vi "Write From File To Instrument.vi"(8 "error in (no error)":errorcluster, 9 "Target Instrument File":string="D:\\user\\data\\test.hcp", 10 "Source PC File":path=path "C:/test.hcp", 11 "VISA resource name":refnum<visa-resource-name>) -> (0 "error out":errorcluster, 3 "VISA resource name out":refnum<visa-resource-name>)   [LabVIEW 2020, in "Rohde&Schwarz CMXP GPRF.lvlib"]
doc: "This VI copies a file from the host computer to the instrument:\n<b>PC FILE -> INSTRUMENT FILE</b>\n\nRemote-control command:\nMMEMory:DATA <file_name>[,<block data>]"
uses:
  <instrlib>/Rohde&Schwarz CMXP GPRF/Rohde&Schwarz CMXP GPRF.lvlib
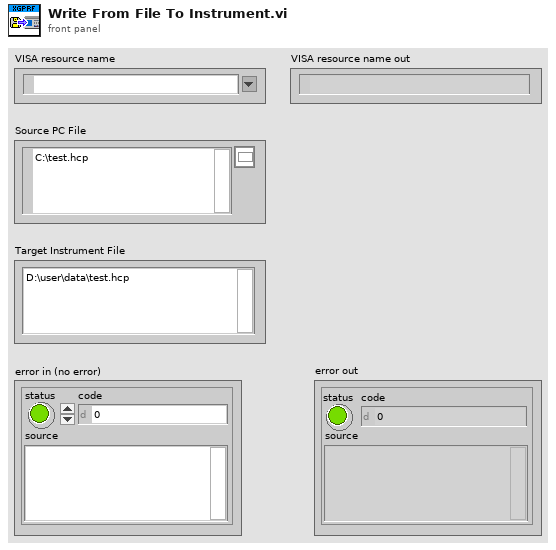
[diagram p1: front panel]
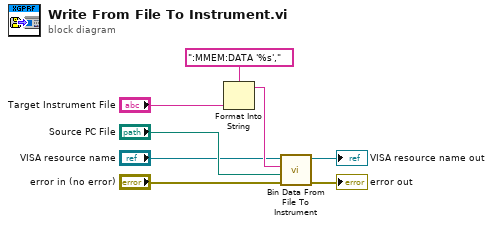
[diagram p0: block diagram]
diagram:
  n1 = Format Into String(format string=":MMEM:DATA '%s',", "Target Instrument File") -> (resulting string=w3:string)  [unwired: 2 in, 1 out]
  n2 = call <instrlib>:"Bin Data From File To Instrument.vi"("error in (no error)"="error in (no error)", "Source PC File"="Source PC File", "Command"=w3, "VISA resource name"="VISA resource name") -> ("error out"=→"error out":errorcluster, "VISA resource name out"=→"VISA resource name out":refnum<visa-resource-name>)  [unwired: 6 in]
